vi "Set Shooter Speed.vi"(10 "Buttons":T2, 11 "Axes":T1) -> (3 "Shooter Speed":dbl)   [LabVIEW 2011]
uses:
  <vilib>/Rock Robotics/WPI/Joystick/WPI_JoystickButtonState.ctl
  Robot Global Data.vi
panel:
  in  "Sonar Trim Factor":dbl(slide) scale=0.0..0.5
  out "number":u32
  in  "Preset Trim Factor":dbl(slide) scale=0.0..0.5
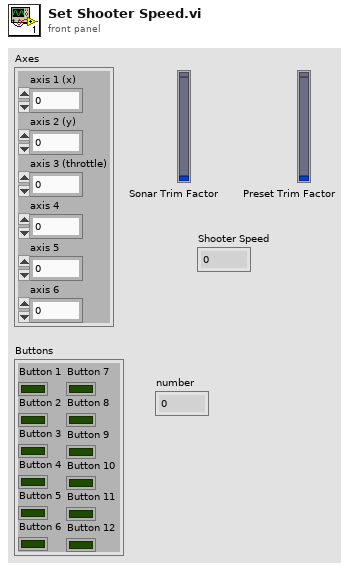
[diagram p1: front panel]
types:
  T1 = cluster{"axis 1 (x)":dbl, "axis 2 (y)":dbl, "axis 3 (throttle)":dbl, "axis 4":dbl, "axis 5":dbl, "axis 6":dbl}
  T2 = typedef "WPI_JoystickButtonState.ctl" = cluster{"Button 1":bool, "Button 2":bool, "Button 3":bool, "Button 4":bool, "Button 5":bool, "Button 6":bool, "Button 7":bool, "Button 8":bool, "Button 9":bool, "Button 10":bool, "Button 11":bool, "Button 12":bool}
  T3 = cluster{"Button 2":bool, "Button 3":bool, "Button 4":bool, "Button 5":bool}
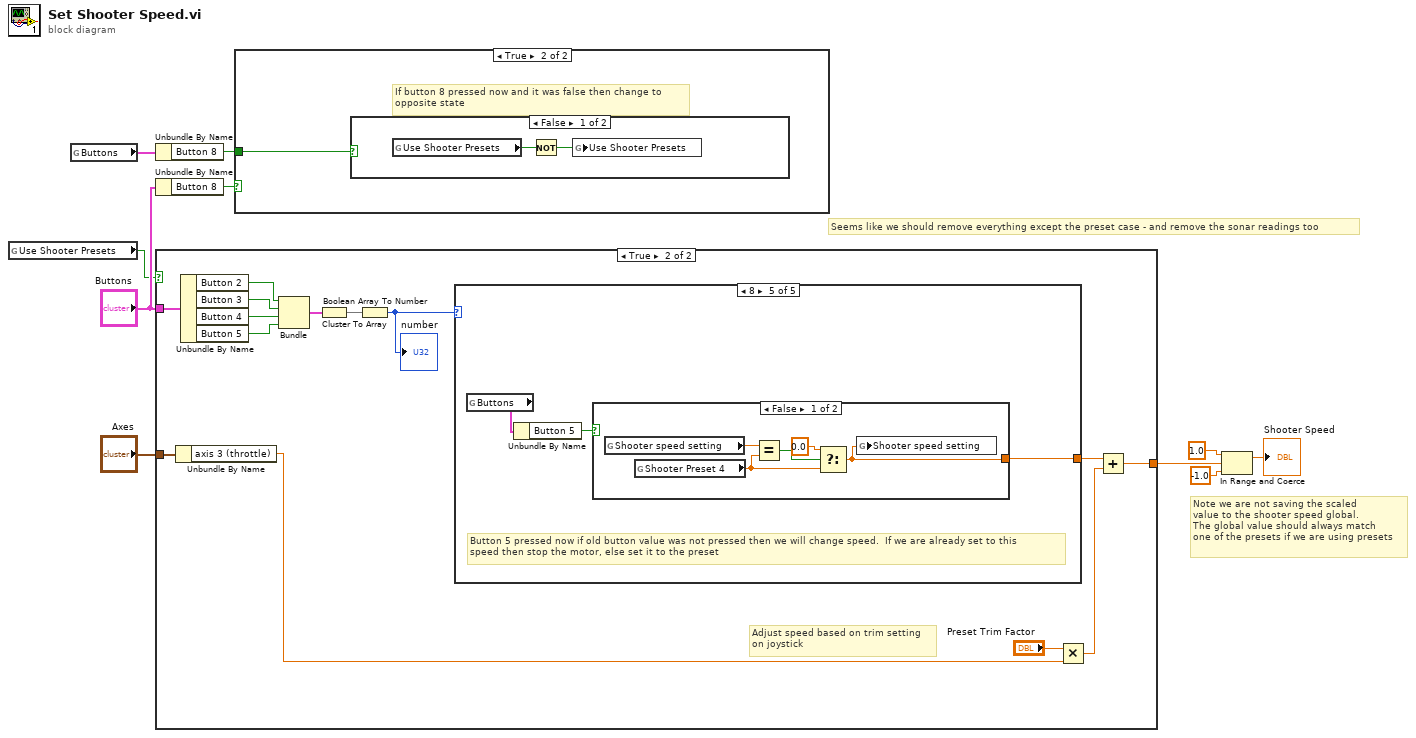
[diagram p0: block diagram]
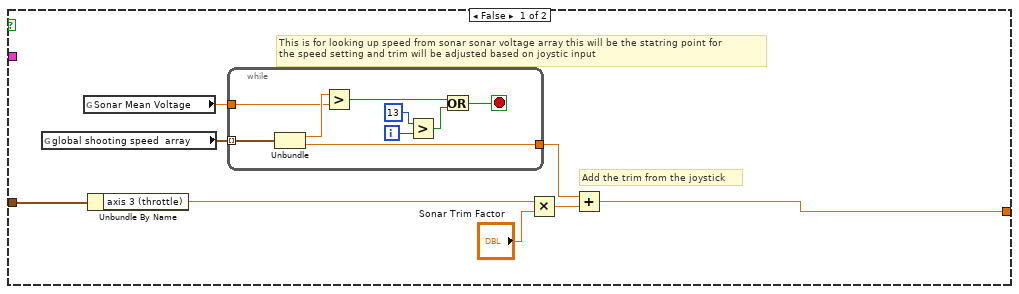
[diagram p4: hidden frame]
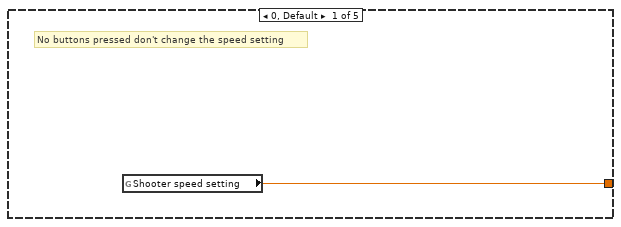
[diagram p5: hidden frame]
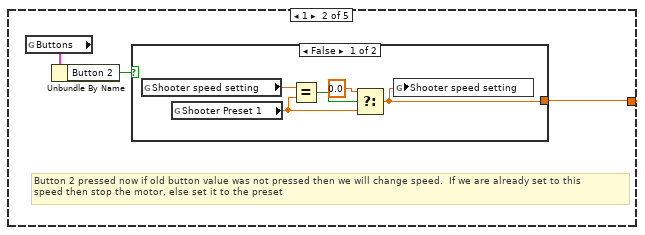
[diagram p6: hidden frame]
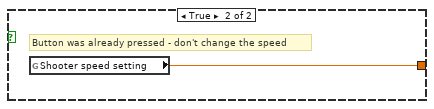
[diagram p7: hidden frame]
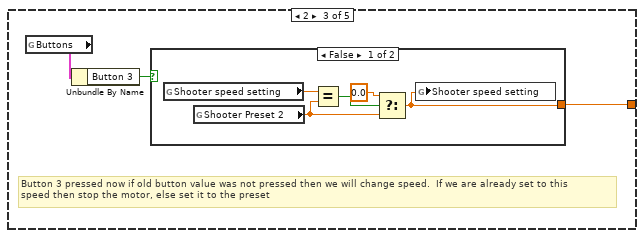
[diagram p8: hidden frame]
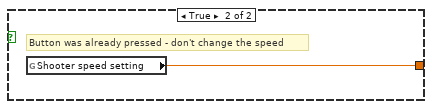
[diagram p9: hidden frame]
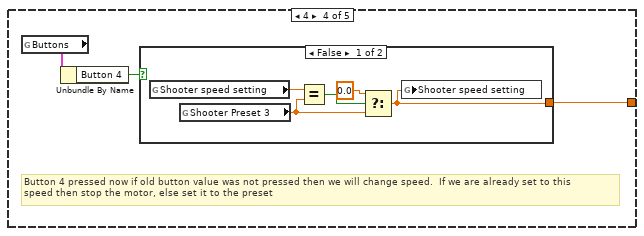
[diagram p10: hidden frame]
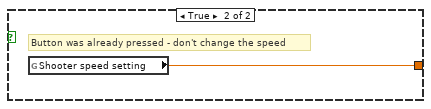
[diagram p11: hidden frame]
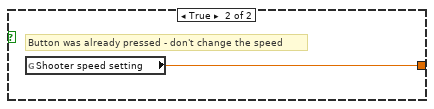
[diagram p12: hidden frame]
diagram:
  # "Seems like we should remove everything except the preset case - and remove the sonar readings too"
  # "Note we are not saving the scaled \nvalue to the shooter speed global.  \nThe global value should always match \none of the presets if we are using presets"
  n1 = global read "Robot Global Data.vi" "Use Shooter Presets"() -> (w7:bool)
  n2 = global read "Robot Global Data.vi" "Buttons"() -> (w8:T2)
  n3 = Unbundle By Name(w8) -> ("Button 8"=w5:bool)
  n4 = Unbundle By Name("Buttons") -> ("Button 8"=w6:bool)
  n5 = case shown="True" w7 {
    tunnel: "Axes" -> [w18 w33]
    tunnel: [w15 w31] -> w2
    tunnel: "Buttons" -> [_ w41]
    frame False {
      # "This is for looking up speed from sonar sonar voltage array this will be the statring point for  \nthe speed setting and trim will be adjusted based on joystic input"
      # "Add the trim from the joystick"
      n6 = global read "Robot Global Data.vi" "global shooting speed  array"() -> (w16:cluster{dbl, dbl}[])
      n7 = global read "Robot Global Data.vi" "Sonar Mean Voltage"() -> (w17:dbl)
      n8 = Unbundle By Name(w18) -> ("axis 3 (throttle)"=w11:dbl)
      n9 = while {
        tunnel: w16 -> [w27] mode=indexing
        tunnel: [w25] -> w14
        tunnel: w17 -> [w24]
        i -> [w23]
        stop <- w19 stop-if-true
        n10 = Unbundle(w27) -> (w26:dbl, w25:dbl)
        n11 = Greater?(x=w26, y=w24) -> (0:w21:bool)
        n12 = Greater?(x=13, y=w23) -> (0:w20:bool)
        n13 = Or(x=w21, y=w20) -> (x .or. y?=w19:bool)
      }
      n14 = Multiply(x=w11, y="Sonar Trim Factor") -> (x*y=w13:dbl)
      n15 = Add(x=w14, y=w13) -> (x+y=w15:dbl)
    }
    frame True {
      # "Adjust speed based on trim setting\non joystick"
      n16 = Unbundle By Name(w33) -> ("axis 3 (throttle)"=w28:dbl)
      n17 = Unbundle By Name(w41) -> ("Button 2"=w40:bool, "Button 3"=w39:bool, "Button 4"=w38:bool, "Button 5"=w37:bool)
      n18 = Bundle("Button 2"=w40, "Button 3"=w39, "Button 4"=w38, "Button 5"=w37) -> (w36:T3)  [unwired: 1 in]
      n19 = Cluster To Array(cluster=w36) -> (array=w35:bool[])
      n20 = Boolean Array To Number(Boolean array=w35) -> (number=w34:u32)
      "number" <- w34
      n21 = case shown="8" w34 {
        tunnel: [w42 w43 w52 w61 w70] -> w30
        frame 0, Default {
          # "No buttons pressed don't change the speed setting"
          n22 = global read "Robot Global Data.vi" "Shooter speed setting"() -> (w42:dbl)
        }
        frame 1 {
          # "Button 2 pressed now if old button value was not pressed then we will change speed.  If we are already set to this \nspeed then stop the motor, else set it to the preset"
          n23 = global read "Robot Global Data.vi" "Buttons"() -> (w45:T2)
          n24 = Unbundle By Name(w45) -> ("Button 2"=w44:bool)
          n25 = case shown="False" w44 {
            tunnel: [w46 w51] -> w43
            frame False {
              n26 = global read "Robot Global Data.vi" "Shooter speed setting"() -> (w49:dbl)
              n27 = global read "Robot Global Data.vi" "Shooter Preset 1"() -> (w48:dbl)
              n28 = Equal?(x=w49, y=w48) -> (x = y?=w50:bool)
              n29 = Select(t=0.0, s=w50, f=w48) -> (s? t:f=w46:dbl)
              n30 = global write "Robot Global Data.vi" "Shooter speed setting"(w46) -> ()
            }
            frame True {
              # "Button was already pressed - don't change the speed"
              n31 = global read "Robot Global Data.vi" "Shooter speed setting"() -> (w51:dbl)
            }
          }
        }
        frame 2 {
          # "Button 3 pressed now if old button value was not pressed then we will change speed.  If we are already set to this \nspeed then stop the motor, else set it to the preset"
          n32 = global read "Robot Global Data.vi" "Buttons"() -> (w54:T2)
          n33 = Unbundle By Name(w54) -> ("Button 3"=w53:bool)
          n34 = case shown="False" w53 {
            tunnel: [w55 w60] -> w52
            frame False {
              n35 = global read "Robot Global Data.vi" "Shooter speed setting"() -> (w58:dbl)
              n36 = global read "Robot Global Data.vi" "Shooter Preset 2"() -> (w57:dbl)
              n37 = Equal?(x=w58, y=w57) -> (x = y?=w59:bool)
              n38 = Select(t=0.0, s=w59, f=w57) -> (s? t:f=w55:dbl)
              n39 = global write "Robot Global Data.vi" "Shooter speed setting"(w55) -> ()
            }
            frame True {
              # "Button was already pressed - don't change the speed"
              n40 = global read "Robot Global Data.vi" "Shooter speed setting"() -> (w60:dbl)
            }
          }
        }
        frame 4 {
          # "Button 4 pressed now if old button value was not pressed then we will change speed.  If we are already set to this \nspeed then stop the motor, else set it to the preset"
          n41 = global read "Robot Global Data.vi" "Buttons"() -> (w63:T2)
          n42 = Unbundle By Name(w63) -> ("Button 4"=w62:bool)
          n43 = case shown="False" w62 {
            tunnel: [w64 w69] -> w61
            frame False {
              n44 = global read "Robot Global Data.vi" "Shooter speed setting"() -> (w67:dbl)
              n45 = global read "Robot Global Data.vi" "Shooter Preset 3"() -> (w66:dbl)
              n46 = Equal?(x=w67, y=w66) -> (x = y?=w68:bool)
              n47 = Select(t=0.0, s=w68, f=w66) -> (s? t:f=w64:dbl)
              n48 = global write "Robot Global Data.vi" "Shooter speed setting"(w64) -> ()
            }
            frame True {
              # "Button was already pressed - don't change the speed"
              n49 = global read "Robot Global Data.vi" "Shooter speed setting"() -> (w69:dbl)
            }
          }
        }
        frame 8 {
          # "Button 5 pressed now if old button value was not pressed then we will change speed.  If we are already set to this \nspeed then stop the motor, else set it to the preset"
          n50 = global read "Robot Global Data.vi" "Buttons"() -> (w72:T2)
          n51 = Unbundle By Name(w72) -> ("Button 5"=w71:bool)
          n52 = case shown="False" w71 {
            tunnel: [w73 w78] -> w70
            frame False {
              n53 = global read "Robot Global Data.vi" "Shooter speed setting"() -> (w76:dbl)
              n54 = global read "Robot Global Data.vi" "Shooter Preset 4"() -> (w75:dbl)
              n55 = Equal?(x=w76, y=w75) -> (x = y?=w77:bool)
              n56 = Select(t=0.0, s=w77, f=w75) -> (s? t:f=w73:dbl)
              n57 = global write "Robot Global Data.vi" "Shooter speed setting"(w73) -> ()
            }
            frame True {
              # "Button was already pressed - don't change the speed"
              n58 = global read "Robot Global Data.vi" "Shooter speed setting"() -> (w78:dbl)
            }
          }
        }
      }
      n59 = Multiply(x="Preset Trim Factor", y=w28) -> (x*y=w29:dbl)
      n60 = Add(x=w30, y=w29) -> (x+y=w31:dbl)
    }
  }
  n61 = case shown="True" w6 {
    tunnel: w5 -> [_ w79]
    frame False {
      # "If button 7 is not press don't change the  value"
    }
    frame True {
      # "If button 8 pressed now and it was false then change to \nopposite state"
      n62 = case shown="False" w79 {
        frame False {
          n63 = global read "Robot Global Data.vi" "Use Shooter Presets"() -> (w81:bool)
          n64 = Not(x=w81) -> (.not. x?=w80:bool)
          n65 = global write "Robot Global Data.vi" "Use Shooter Presets"(w80) -> ()
        }
        frame True {
        }
      }
    }
  }
  n66 = In Range and Coerce(upper limit=1.0, x=w2, lower limit=-1.0) -> (coerced(x)=→"Shooter Speed":dbl)  [unwired: 1 out]
